vi "Set Step Name.vi"(8 "error in (no error)":errorcluster, 10 "Standard":string, 11 "Servo to Power Out in":refnum<class "Servo to Power Out.lvclass">) -> (0 "error out":errorcluster, 2 "Step Name":string, 3 "Servo to Power Out out":refnum<class "Servo to Power Out.lvclass">)   [LabVIEW 2018, in "Servo to Power Out.lvlib" / "Servo to Power Out.lvclass"]
uses:
  Servo to Power Out.lvclass
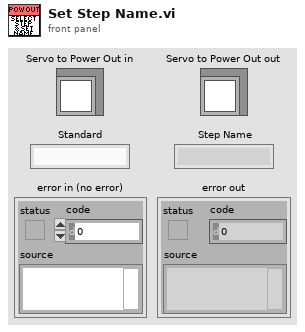
[diagram p1: front panel]
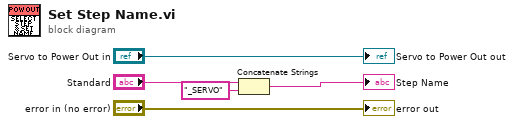
[diagram p0: block diagram]
diagram:
  n1 = Concatenate Strings("Standard", "_SERVO" ("string")) -> (→"Step Name":string)
  "error out" <- "error in (no error)"
  "Servo to Power Out out" <- "Servo to Power Out in"
